vi "TRITON_PARSE_VECTOR.vi"(0 "String":string) -> (1 "X":dbl, 2 "Y":dbl, 3 "Z":dbl)   [LabVIEW 2009]
panel:
  out "Z":string
  out "Y":string
  out "X":string
  out "index of end element":i32
  out "index of start element":i32
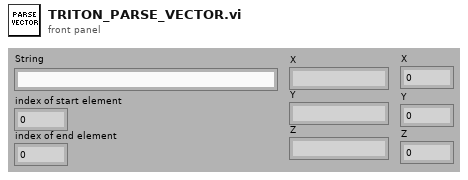
[diagram p1: front panel]
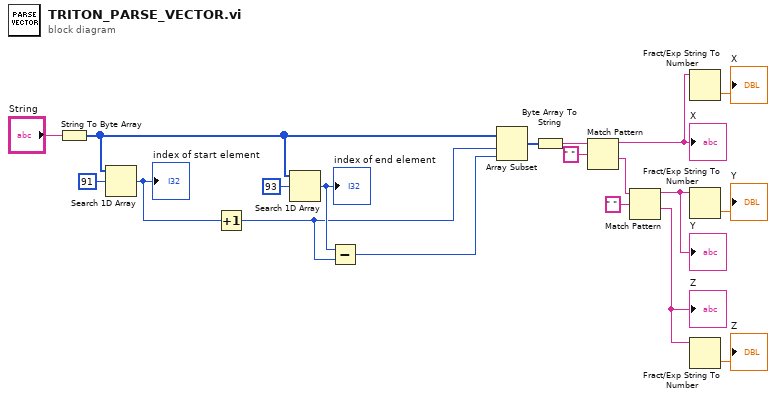
[diagram p0: block diagram]
diagram:
  n1 = String To Byte Array(string="String") -> (unsigned byte array=w16:u8[])
  n2 = Search 1D Array(1D array=w16, element=u8 91) -> (index of element=w12:i32)  [unwired: 1 in]
  "index of start element" <- w12
  n3 = Increment(x=w12) -> (x+1=w11:i32)
  n4 = Search 1D Array(1D array=w16, element=u8 93) -> (index of element=w15:i32)  [unwired: 1 in]
  "index of end element" <- w15
  n5 = Subtract(x=w15, y=w11) -> (x-y=w14:i32)
  n6 = Array Subset(array=w16, index=w11, length=w14) -> (w13:u8[])
  n7 = Byte Array To String(unsigned byte array=w13) -> (string=w10:string)
  n8 = Match Pattern(string=w10, regular expression=" ") -> (before substring=w6:string, after substring=w7:string)  [unwired: 1 in, 2 out]
  "X" <- w6
  n9 = Match Pattern(string=w7, regular expression=" ") -> (before substring=w4:string, after substring=w5:string)  [unwired: 1 in, 2 out]
  "Y" <- w4
  "Z" <- w5
  n10 = Fract/Exp String To Number(string=w6) -> (number=→"X":dbl)  [unwired: 3 in, 1 out]
  n11 = Fract/Exp String To Number(string=w4) -> (number=→"Y":dbl)  [unwired: 3 in, 1 out]
  n12 = Fract/Exp String To Number(string=w5) -> (number=→"Z":dbl)  [unwired: 3 in, 1 out]
